vi "Script Module Timeout.vi"(5 "Restore to Default":bool, 7 "Theme":bool, 8 "error in":errorcluster, 10 "Library in":refnum<vi>, 11 "App Ref":refnum<vi>) -> (0 "error out":errorcluster)   [LabVIEW 2019, in "Panther Dashboard.lvlib"]
uses:
  Panther Dashboard.lvlib
  <vilib>/Utility/traverseref.llb/TRef TravTarget.ctl
  <vilib>/Utility/traverseref.llb/VI Scripting - Traverse.lvlib
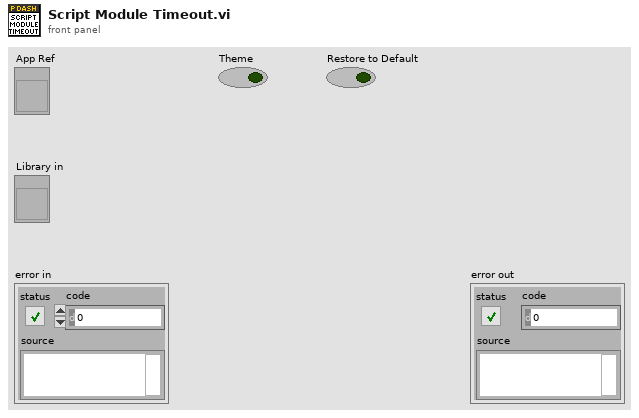
[diagram p1: front panel]
types:
  T1 = typedef "TRef TravTarget.ctl" = enum16{"FP", "BD", "Other"}
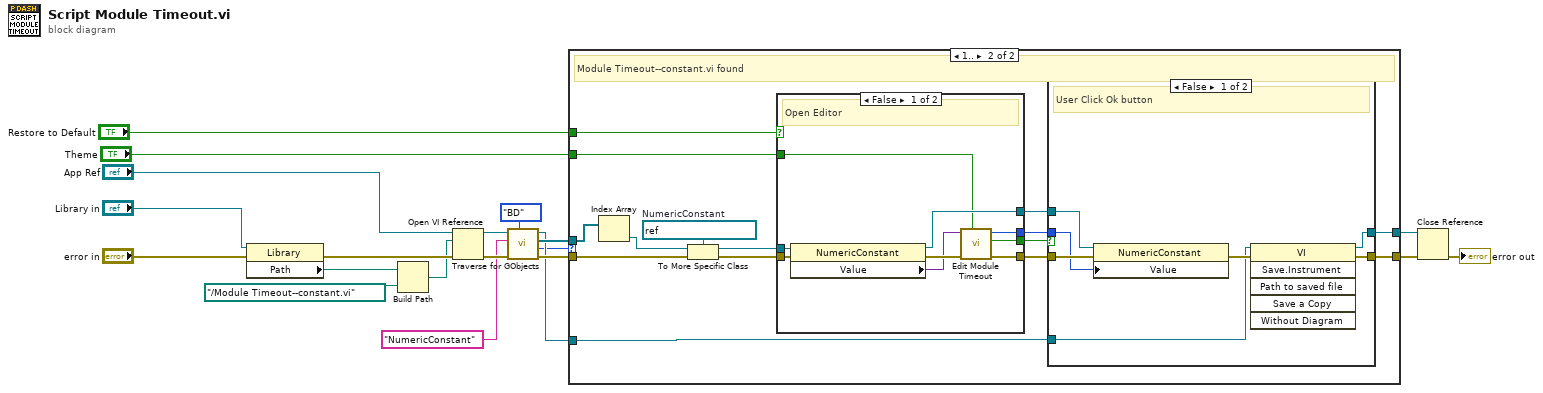
[diagram p0: block diagram]
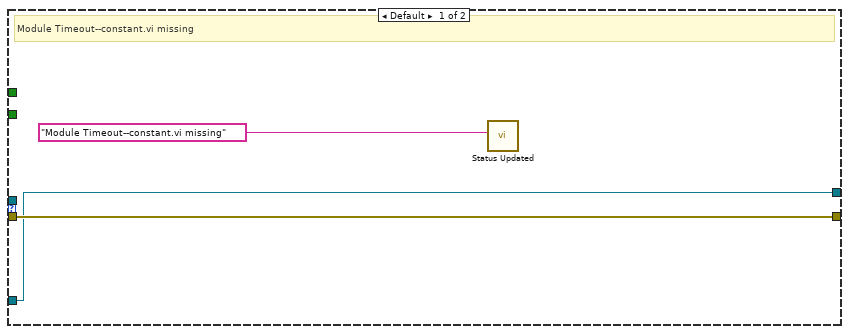
[diagram p2: hidden frame]
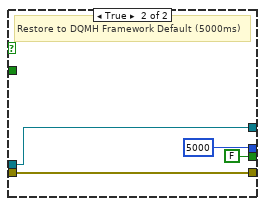
[diagram p3: hidden frame]
diagram:
  n1 = property class="Library"(reference="Library in", error in="error in") -> (error out=w19:errorcluster, "Path"=w13:path)  [unwired: 1 out]
  n2 = Build Path(base path=w13, name or relative path=path "../Module Timeout--constant.vi") -> (appended path=w11:path)
  n3 = Open VI Reference(application reference (local)="App Ref", vi path=w11, error in (no error)=w19) -> (vi reference=w9:refnum<vi>, error out=w18:errorcluster)  [unwired: 3 in]
  n4 = call <vilib>:"Traverse for GObjects.vi"("Traverse Target"=TRef_TravTarget."BD", "error in (no error)"=w18, "Class Name"="NumericConstant", "VI Refnum"=w9) -> ("error out"=w17:errorcluster, "# of Refs"=w2:i32, "References"=w6:refnum<vi>[], "dup VI Refnum"=w4:refnum<vi>)  [unwired: 4 in]
  n5 = case shown="1.." w2 {
    tunnel: w17 -> [w23 w38]
    tunnel: w6 -> [_ w26]
    tunnel: "Theme" -> [_ w29]
    tunnel: w4 -> [w21 w28]
    tunnel: [w21 w27] -> w3
    tunnel: [w23 w35] -> w15
    tunnel: "Restore to Default" -> [_ w24]
    frame Default {
      # "Module Timeout--constant.vi missing"
      n6 = call "Status Updated.vi"("Status"="Module Timeout--constant.vi missing") -> ()  [unwired: 10 in, 1 out]
    }
    frame 1.. {
      w34 = refnum<vi> refnum  # NumericConstant
      # "Module Timeout--constant.vi found"
      n7 = Index Array(array=w26) -> (element=w25:refnum<vi>)  [unwired: 1 in]
      n8 = To More Specific Class(target class=w34, reference=w25, error in=w38) -> (specific class reference=w33:refnum<vi>, error out=w37:errorcluster)
      n9 = case shown="False" w24 {
        tunnel: w37 -> [w47 w51]
        tunnel: [w45 w51] -> w36
        tunnel: w33 -> [w44 w50]
        tunnel: [w42 w50] -> w32
        tunnel: [w41 5000 ("New Module Timeout")] -> w31
        tunnel: [w40 FALSE ("Canceled")] -> w30
        tunnel: w29 -> [w39 _]
        frame False {
          # "Open Editor"
          n10 = property class="NumericConstant"(reference=w44, error in=w47) -> (reference out=w42:refnum<vi>, error out=w46:errorcluster, "Value"=w43:variant)
          n11 = call "Edit Module Timeout.vi"("Theme"=w39, "error in"=w46, "Value"=w43) -> ("error out"=w45:errorcluster, "Canceled"=w40:bool, "New Module Timeout"=w41:i32)  [unwired: 6 in]
        }
        frame True {
          # "Restore to DQMH Framework Default (5000ms)"
        }
      }
      n12 = case shown="False" w30 {
        tunnel: w36 -> [w58 w60]
        tunnel: w32 -> [w55 _]
        tunnel: w31 -> [w54 _]
        tunnel: w28 -> [w53 w59]
        tunnel: [w52 w59] -> w27
        tunnel: [w57 w60] -> w35
        frame False {
          # "User Click Ok button"
          n13 = property class="NumericConstant"(reference=w55, error in=w58, "Value"=w54) -> (error out=w56:errorcluster)  [unwired: 1 out]
          n14 = invoke class="VI" method="Save.Instrument"(reference=w53, error in=w56) -> (reference out=w52:refnum<vi>, error out=w57:errorcluster)  [unwired: 4 in, 4 out]
        }
        frame True {
          # "User Cancel"
        }
      }
    }
  }
  n15 = Close Reference(reference=w3, error in (no error)=w15) -> (error out=→"error out":errorcluster)
